vi "Get Pad Transform.vi"(8 "error in (no error)":errorcluster, 9 "Length Z":sgl, 10 "Key Points":dbl[](array[numeric]), 11 "position on path":dbl) -> (0 "error out":errorcluster, 2 "angle":dbl, 3 "translation":cluster{"X":sgl, "Y":sgl, "Z":sgl})   [LabVIEW 2017, in "NI_Robotics_Simulator.lvlib" / "ODESimulator_LinearConveyor.lvclass"]
uses:
  <vilib>/robotics/Simulator/Robot Factory/Conveyor/Linear/ODESimulator_LinearConveyor.lvclass
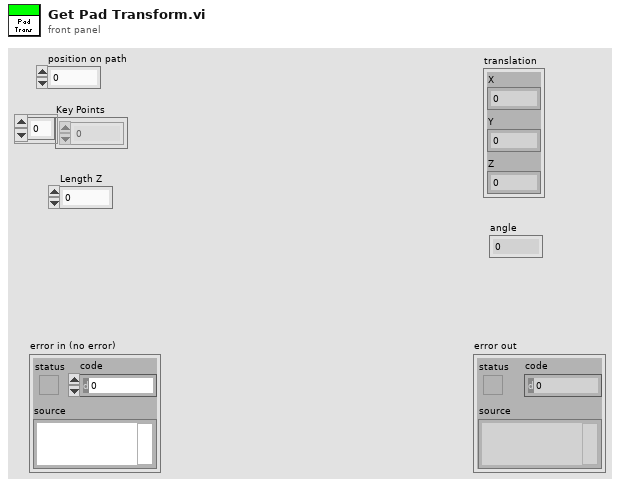
[diagram p1: front panel]
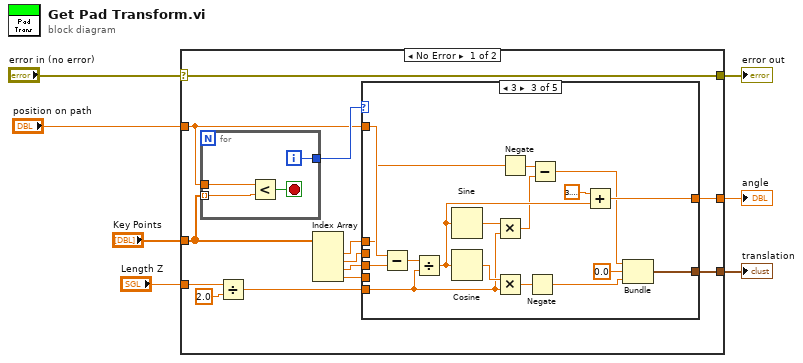
[diagram p0: block diagram]
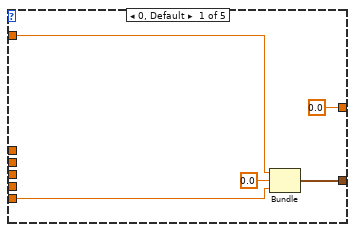
[diagram p2: hidden frame]
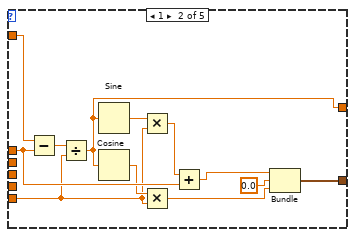
[diagram p3: hidden frame]
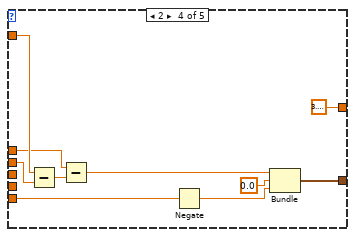
[diagram p4: hidden frame]
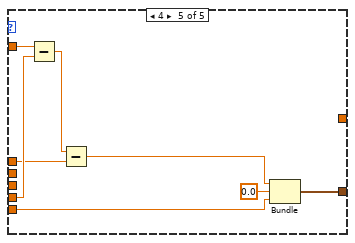
[diagram p5: hidden frame]
diagram:
  n1 = case shown="No Error" "error in (no error)" {
    selector: "error in (no error)" -> [w20 w77]
    tunnel: [w20 w77] -> w6
    tunnel: "position on path" -> [w10 _]
    tunnel: [w12 _] -> w4
    tunnel: [w11 _] -> w3
    tunnel: "Key Points" -> [w9 _]
    tunnel: "Length Z" -> [w8 _]
    frame No Error {
      n2 = for {
        tunnel: w9 -> [w76] mode=indexing
        tunnel: [w74] -> w19
        tunnel: w10 -> [w73]
        i -> [w74]
        stop <- w75 stop-if-true
        n3 = Less?(x=w73, y=w76) -> (x < y?=w75:bool)
      }
      n4 = Divide(x=w8, y=sgl 2.0) -> (x/y=w13:sgl)
      n5 = Index Array(array=w9) -> (element #1=w18:dbl, element #2=w17:dbl, element #3=w16:dbl, element #4=w15:dbl)  [unwired: 4 in]
      n6 = case shown="3" w19 {
        tunnel: w10 -> [w25 w37 w54 w64 w72]
        tunnel: w13 -> [w23 w32 w50 w58 w66]
        tunnel: [w22 w27 w48 w56 w65] -> w12
        tunnel: [0.0 w26 w43 3.141592653589793 _] -> w11
        tunnel: w18 -> [_ w35 w41 w61 w69]
        tunnel: w17 -> [_ _ _ w63 _]
        tunnel: w16 -> [_ _ w47 _ _]
        tunnel: w15 -> [_ _ _ _ w71]
        frame 0, Default {
          n7 = Bundle("position on path"=w25, 0.0, w23) -> (w22:cluster{"position on path":dbl, dbl, sgl})  [unwired: 1 in]
        }
        frame 1 {
          n8 = Subtract(x=w37, y=w35) -> (x-y=w36:dbl)
          n9 = Divide(x=w36, y=w32) -> (x/y=w26:dbl)
          n10 = Sine(x=w26) -> (sin(x)=w34:dbl)
          n11 = Cosine(x=w26) -> (cos(x)=w33:dbl)
          n12 = Multiply(x=w34, y=w32) -> (x*y=w31:dbl)
          n13 = Multiply(x=w33, y=w32) -> (x*y=w28:dbl)
          n14 = Add(x=w31, y=w35) -> (x+y=w30:dbl)
          n15 = Bundle(w30, 0.0, w28) -> (w27:cluster{dbl, dbl, dbl})  [unwired: 1 in]
        }
        frame 3 {
          n16 = Subtract(x=w54, y=w47) -> (x-y=w53:dbl)
          n17 = Divide(x=w53, y=w50) -> (x/y=w44:dbl)
          n18 = Sine(x=w44) -> (sin(x)=w52:dbl)
          n19 = Cosine(x=w44) -> (cos(x)=w51:dbl)
          n20 = Multiply(x=w52, y=w50) -> (x*y=w39:dbl)
          n21 = Multiply(x=w51, y=w50) -> (x*y=w46:dbl)
          n22 = Negate(x=w41) -> (-x=w40:dbl)
          n23 = Negate(x=w46) -> (-x=w45:dbl)
          n24 = Subtract(x=w40, y=w39) -> (x-y=w38:dbl)
          n25 = Add(x=3.141592653589793, y=w44) -> (x+y=w43:dbl)
          n26 = Bundle(w38, 0.0, w45) -> (w48:cluster{dbl, dbl, dbl})  [unwired: 1 in]
        }
        frame 2 {
          n27 = Subtract(x=w64, y=w63) -> (x-y=w62:dbl)
          n28 = Subtract(x=w61, y=w62) -> (x-y=w60:dbl)
          n29 = Negate(x=w58) -> (-x=w57:sgl)
          n30 = Bundle(w60, 0.0, w57) -> (w56:cluster{dbl, dbl, sgl})  [unwired: 1 in]
        }
        frame 4 {
          n31 = Subtract(x=w72, y=w71) -> (x-y=w70:dbl)
          n32 = Subtract(x=w70, y=w69) -> (x-y=w68:dbl)
          n33 = Bundle(w68, 0.0, w66) -> (w65:cluster{dbl, dbl, sgl})  [unwired: 1 in]
        }
      }
    }
    frame Error {
    }
  }
  "error out" <- w6
  "translation" <- w4
  "angle" <- w3
